vi "Get Data Folder.vi"() -> (3 "Data Folder Path":path)   [LabVIEW 2019, in "Project.Dependencies Finder.lvlib"]
doc: "Returns path to the data folder. Assumes PPL is loaded from the data folder."
uses:
  Project.Dependencies Finder.lvlib
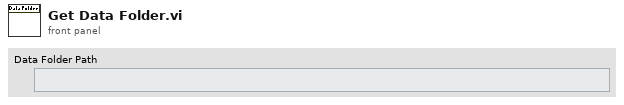
[diagram p1: front panel]
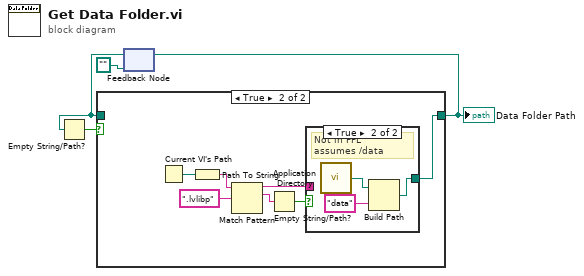
[diagram p0: block diagram]
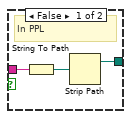
[diagram p3: hidden frame]
diagram:
  n1 = feedback #1(path "") -> (w1:path)
  n2 = Empty String/Path?(string/path=w1) -> (empty?=w3:bool)
  n3 = case shown="True" w3 {
    tunnel: [w5 w12] -> w2
    tunnel: w1 -> [w5 _]
    frame False {
    }
    frame True {
      n4 = Current VI's Path() -> (path=w11:path)
      n5 = Path To String(path=w11) -> (string=w10:string)
      n6 = Match Pattern(string=w10, regular expression=".lvlibp") -> (before substring=w8:string, match substring=w7:string)  [unwired: 1 in, 2 out]
      n7 = Empty String/Path?(string/path=w7) -> (empty?=w6:bool)
      n8 = case shown="True" w6 {
        tunnel: [w15 w16] -> w12
        tunnel: w8 -> [w14 _]
        frame False {
          # "In PPL"
          n9 = String To Path(string=w14) -> (path=w13:path)
          n10 = Strip Path(path=w13) -> (stripped path=w15:path)  [unwired: 1 out]
        }
        frame True {
          # "Not in PPL assumes /data"
          n11 = call <vilib>:"Application Directory.vi"() -> ("Application Directory"=w18:path)
          n12 = Build Path(base path=w18, name or relative path="data") -> (appended path=w16:path)
        }
      }
    }
  }
  "Data Folder Path" <- w2
  n13 = feedback-in #1(w2) -> ()
